vi "Create.vi"(8 "error in":errorcluster, 11 "Reference":refnum<vi>) -> (0 "error out":errorcluster, 3 "Selector out":refnum<class "Selector.lvclass">)   [LabVIEW 2019, in "Selector.lvclass"]
uses:
  Selector.lvclass
  Item.ctl
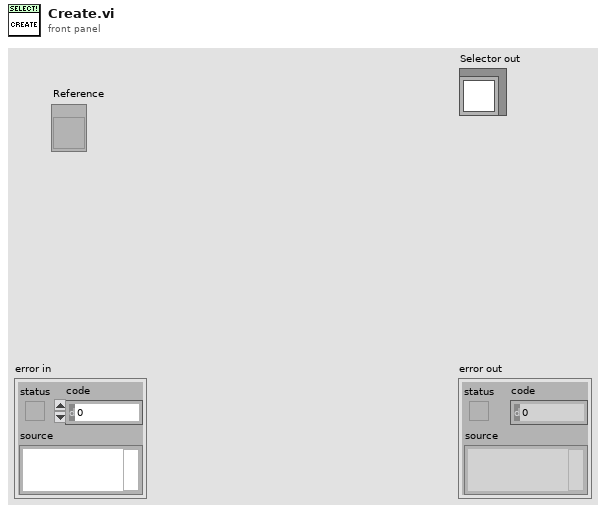
[diagram p1: front panel]
types:
  T1 = typedef "Selector.lvclass/Item.ctl" = cluster{"Name":string, "Group":string, "Enabled":bool}
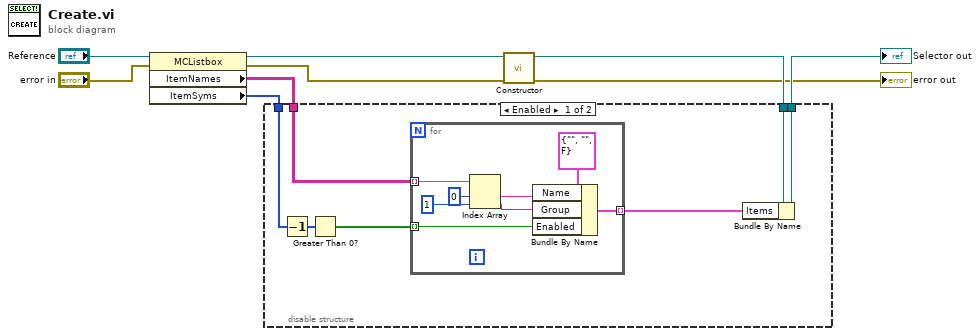
[diagram p0: block diagram]
diagram:
  n1 = property class="MCListbox"(reference="Reference", error in="error in") -> (reference out=w5:refnum<vi>, error out=w1:errorcluster, "ItemNames"=w6:string[][], "ItemSyms"=w8:i32[])
  n2 = call "Constructor.vi"("error in (no error)"=w1, "Reference"=w5) -> ("error out"=→"error out":errorcluster, "MCLB"=w4:refnum<class "Selector.lvclass">)  [unwired: 8 in]
  n3 = disable-structure shown="Enabled" {
    disable-tunnel: w8 -> [w16 _]
    disable-tunnel: w6 -> [w12 _]
    disable-tunnel: w4 -> [w11 w25]
    disable-tunnel: [w10 w25] -> w3
    frame Enabled {
      n4 = Decrement(x=w16) -> (x-1=w14:i32[])
      n5 = Greater Than 0?(x=w14) -> (x > 0?=w15:bool[])
      n6 = for {
        tunnel: w12 -> [w23] mode=indexing
        tunnel: w15 -> [w21] mode=indexing
        tunnel: [w20] -> w13 mode=indexing
        n7 = Index Array(array=w23, index #1=0 ("index"), index #2=1 ("index")) -> (element #1=w22:string, element #2=w17:string)
        n8 = Bundle By Name(cluster=T1 {"Name"="", "Group"="", "Enabled"=FALSE} ("Item"), "Name"=w22, "Group"=w17, "Enabled"=w21) -> (w20:T1)
      }
      n9 = Bundle By Name(cluster=w11, "Items"=w13) -> (w10:refnum<class "Selector.lvclass">)
    }
    frame Disabled {
    }
  }
  "Selector out" <- w3
